vi "Clone Registration AE.vi"(0 "Module ID":i32=-1, 1 "Action":T1=enum."Add Instance", 11 "error in":errorcluster) -> (2 "empty":bool, 3 "Instances Names":string[](array[string]), 4 "Module IDs":i32[](array[numeric]), 6 "First Module ID":i32, 8 "replaced":bool, 10 "Found?":bool, 13 "First?":bool, 14 "First? (all)":bool[](array[boolean]), 15 "error out":errorcluster)   [LabVIEW 2020, in "Arduino stepper.lvlib" / "Clone Registration.lvlib"]
doc: "A registry (implemented as an Action Engine) to store all cloneable module instances. The Action Engine data is stored in a variant attribute table.\n\nOutput <b>First? </b> : We care which module instance was the first as the lifetime of the event references is bound to the lifetime of the module that created them (ie the first module instance). To avoid event references going bad we keep track of the first module and do not close it until safe to do so (ie when all other instances have closed).\n\nIf the first instance is closed whilst others are still running we effectively set that instance to idle. We deregister for all requests except STOP ALL.\n_____\nBased on DQMH Project Template 6.1.0.94."
uses:
  Clone Registration.lvlib
  Action--enum.ctl
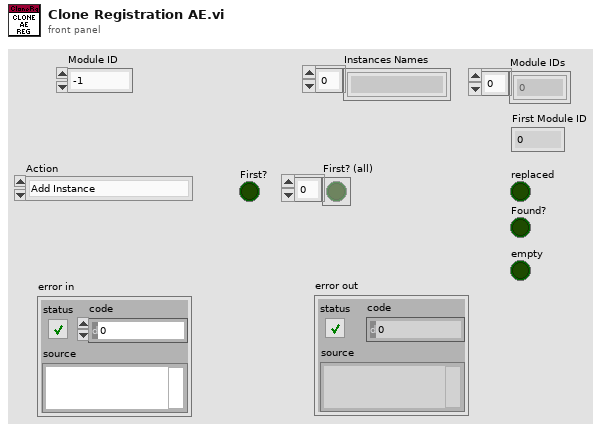
[diagram p1: front panel]
types:
  T1 = typedef "Arduino stepper.lvlib/Clone Registration.lvlib/Action--enum.ctl" = enum16{"Init", "Add Instance", "Remove Instance", "List Instances", "Is First?"}
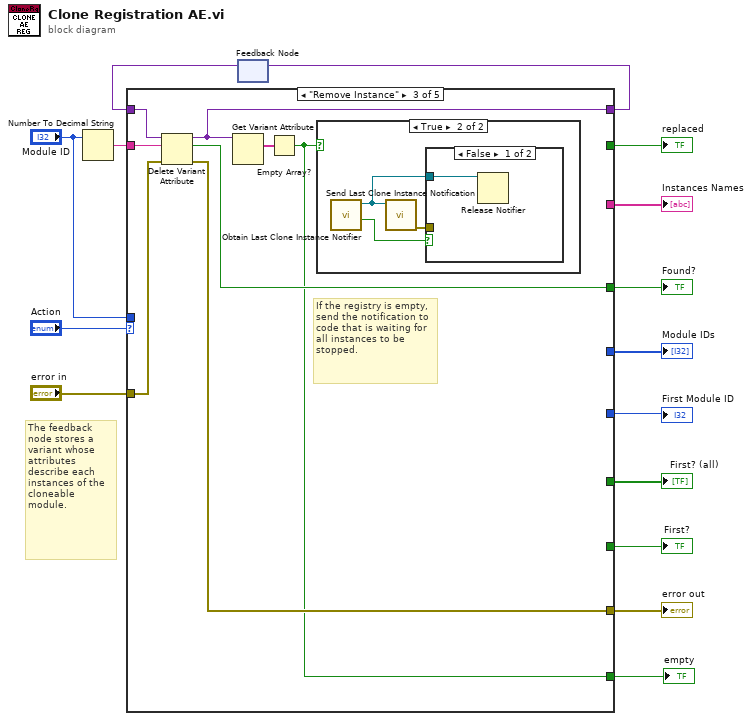
[diagram p0: block diagram]
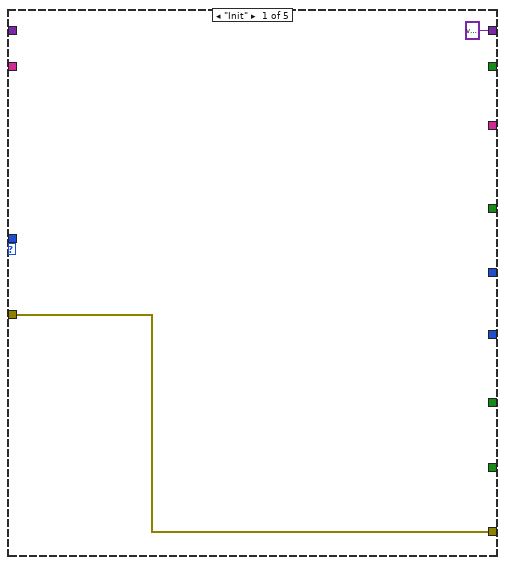
[diagram p2: hidden frame]
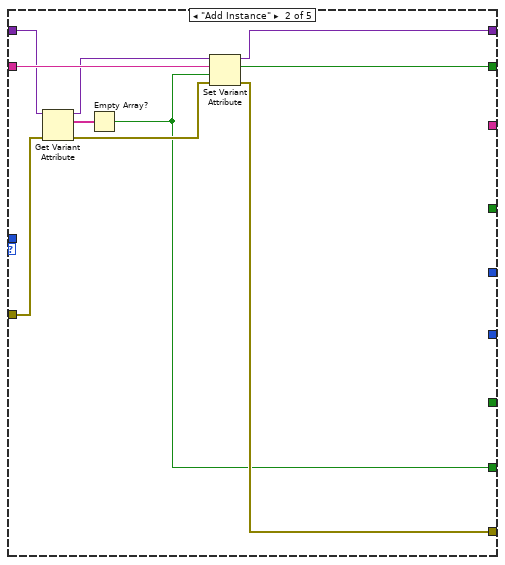
[diagram p3: hidden frame]
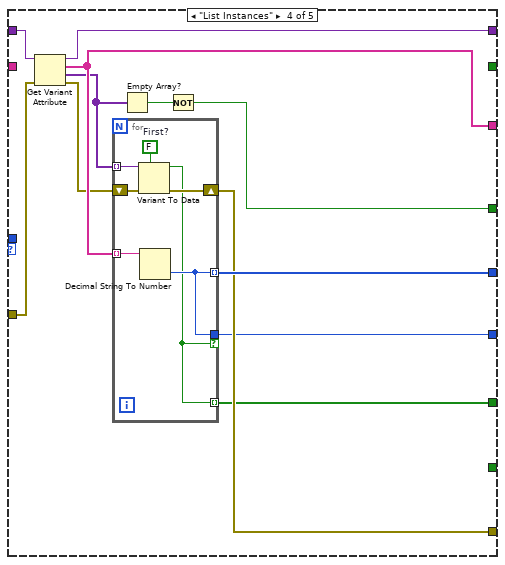
[diagram p6: hidden frame]
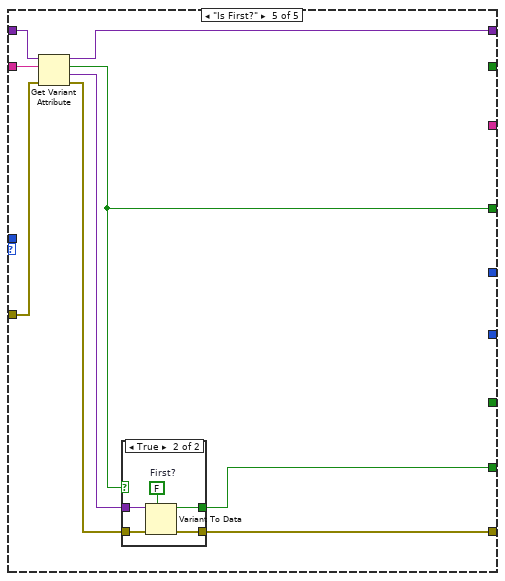
[diagram p7: hidden frame]
diagram:
  # "The feedback node stores a variant whose attributes describe each instances of the cloneable module."
  n1 = Number To Decimal String(number="Module ID") -> (decimal integer string=w14:string)  [unwired: 1 in]
  n2 = feedback #1() -> (w12:variant)  [unwired: 1 in]
  n3 = case shown="\"Remove Instance\"" "Action" {
    tunnel: w12 -> [_ w24 w35 w51 w67]
    tunnel: [variant w27 w30 w50 w66] -> w11
    tunnel: w14 -> [_ w26 w34 _ w61]
    tunnel: [_ w25 _ _ _] -> w10
    tunnel: [_ _ w33 w48 w59] -> w9
    tunnel: "Module ID" -> [_ _ _ _ _]
    tunnel: [_ _ _ w47 _] -> w8
    tunnel: [_ _ _ w46 _] -> w7
    tunnel: [_ _ _ w41 _] -> w6
    tunnel: "error in" -> [w16 w21 w32 w44 w64]
    tunnel: [w16 w19 w31 w42 w62] -> w4
    tunnel: [_ _ _ w40 _] -> w3
    tunnel: [_ w18 _ _ w60] -> w2
    tunnel: [_ _ w28 _ _] -> w1
    frame "Init" {
    }
    frame "Add Instance" {
      n4 = Get Variant Attribute(Variant=w24, error in=w21) -> (duplicate Variant=w23:variant, names=w22:string[], error out=w20:errorcluster)  [unwired: 2 in, 1 out]
      n5 = Empty Array?(array=w22) -> (empty?=w18:bool)
      n6 = Set Variant Attribute(Variant=w23, name=w26, value=w18, error in=w20) -> (Variant out=w27:variant, replaced=w25:bool, error out=w19:errorcluster)
    }
    frame "Remove Instance" {
      # "If the registry is empty, send the notification to code that is waiting for all instances to be stopped."
      n7 = Delete Variant Attribute(4:w32, 6:w34, 7:w35) -> (0:w31:errorcluster, 2:w33:bool, 3:w30:variant)
      n8 = Get Variant Attribute(Variant=w30) -> (names=w29:string[])  [unwired: 3 in, 3 out]
      n9 = Empty Array?(array=w29) -> (empty?=w28:bool)
      n10 = case shown="True" w28 {
        frame False {
        }
        frame True {
          n11 = call "Obtain Last Clone Instance Notifier.vi"() -> ("created new?"=w37:bool, "Last Instance Notifier"=w38:refnum<notifier>)  [unwired: 10 in]
          n12 = call "Send Last Clone Instance Notification.vi"("Last Instance Notifier"=w38) -> ("error out"=w36:errorcluster)  [unwired: 10 in]
          n13 = case shown="False" w37 {
            tunnel: w38 -> [w39 _]
            tunnel: w36 -> [_ _]
            frame False {
              n14 = Release Notifier(notifier=w39) -> ()  [unwired: 2 in, 3 out]
            }
            frame True {
            }
          }
        }
      }
    }
    frame "List Instances" {
      n15 = Get Variant Attribute(Variant=w51, error in=w44) -> (duplicate Variant=w50:variant, names=w46:string[], values=w45:variant[], error out=w43:errorcluster)  [unwired: 2 in]
      n16 = for {
        tunnel: w46 -> [w58] mode=indexing
        tunnel: [w53] -> w47 mode=indexing
        tunnel: w45 -> [w57] mode=indexing
        shift-right: [w54] -> w42
        shift-left: w43 -> [w55]
        tunnel: [w52] -> w41 mode=indexing
        tunnel: [w53] -> w40 if=w52
        w56 = FALSE  # First?
        n17 = Variant To Data(error in=w55, type=w56, Variant=w57) -> (data=w52:bool, error out=w54:errorcluster)
        n18 = Decimal String To Number(string=w58) -> (number=w53:i32)  [unwired: 2 in, 1 out]
      }
      n19 = Empty Array?(array=w45) -> (empty?=w49:bool)
      n20 = Not(x=w49) -> (.not. x?=w48:bool)
    }
    frame "Is First?" {
      n21 = Get Variant Attribute(Variant=w67, name=w61, error in=w64) -> (duplicate Variant=w66:variant, found=w59:bool, value=w65:variant, error out=w63:errorcluster)  [unwired: 1 in]
      n22 = case shown="True" w59 {
        tunnel: w65 -> [_ w73]
        tunnel: w63 -> [w68 w72]
        tunnel: [w68 w71] -> w62
        tunnel: [_ w69] -> w60
        frame False {
        }
        frame True {
          w70 = FALSE  # First?
          n23 = Variant To Data(error in=w72, type=w70, Variant=w73) -> (data=w69:bool, error out=w71:errorcluster)
        }
      }
    }
  }
  "replaced" <- w10
  "Found?" <- w9
  "Module IDs" <- w8
  "Instances Names" <- w7
  "First? (all)" <- w6
  "error out" <- w4
  "First Module ID" <- w3
  "First?" <- w2
  "empty" <- w1
  n24 = feedback-in #1(w11) -> ()
